vi "LV String to Str64.vi"(11 "string":string) -> (3 "str64":T1)   [LabVIEW 2026, in "MrcLib.lvlib"]
uses:
  MrcLib.lvlib
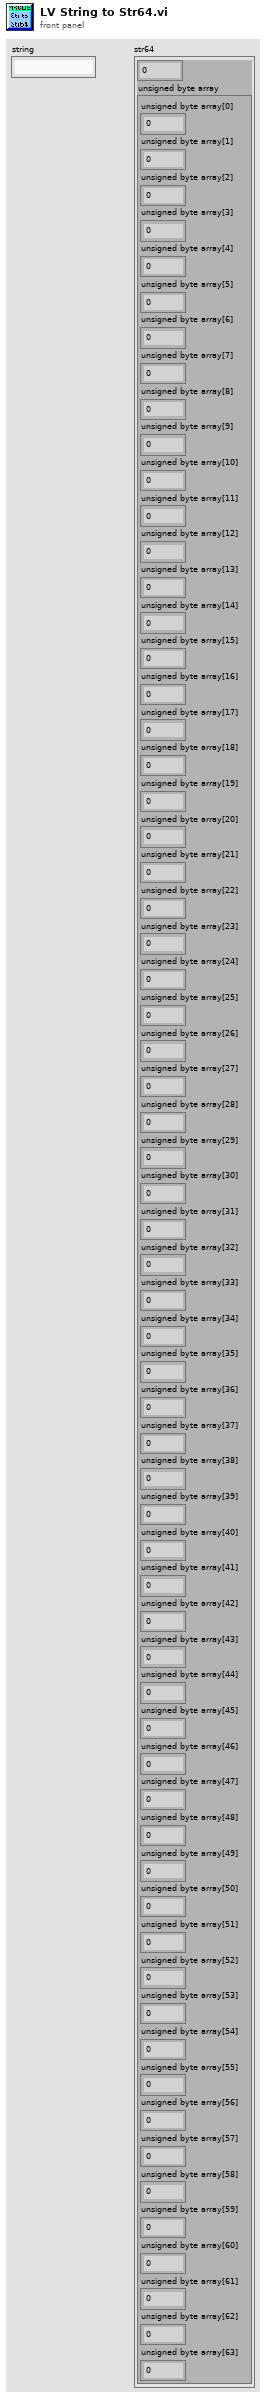
[diagram p1: front panel]
types:
  T1 = cluster{u8, "unsigned byte array":cluster{"unsigned byte array[0]":u8, "unsigned byte array[1]":u8, "unsigned byte array[2]":u8, "unsigned byte array[3]":u8, "unsigned byte array[4]":u8, "unsigned byte array[5]":u8, "unsigned byte array[6]":u8, "unsigned byte array[7]":u8, "unsigned byte array[8]":u8, "unsigned byte array[9]":u8, "unsigned byte array[10]":u8, "unsigned byte array[11]":u8, "unsigned byte array[12]":u8, "unsigned byte array[13]":u8, "unsigned byte array[14]":u8, "unsigned byte array[15]":u8, "unsigned byte array[16]":u8, "unsigned byte array[17]":u8, "unsigned byte array[18]":u8, "unsigned byte array[19]":u8, "unsigned byte array[20]":u8, "unsigned byte array[21]":u8, "unsigned byte array[22]":u8, "unsigned byte array[23]":u8, "unsigned byte array[24]":u8, "unsigned byte array[25]":u8, "unsigned byte array[26]":u8, "unsigned byte array[27]":u8, "unsigned byte array[28]":u8, "unsigned byte array[29]":u8, "unsigned byte array[30]":u8, "unsigned byte array[31]":u8, "unsigned byte array[32]":u8, "unsigned byte array[33]":u8, "unsigned byte array[34]":u8, "unsigned byte array[35]":u8, "unsigned byte array[36]":u8, "unsigned byte array[37]":u8, "unsigned byte array[38]":u8, "unsigned byte array[39]":u8, "unsigned byte array[40]":u8, "unsigned byte array[41]":u8, "unsigned byte array[42]":u8, "unsigned byte array[43]":u8, "unsigned byte array[44]":u8, "unsigned byte array[45]":u8, "unsigned byte array[46]":u8, "unsigned byte array[47]":u8, "unsigned byte array[48]":u8, "unsigned byte array[49]":u8, "unsigned byte array[50]":u8, "unsigned byte array[51]":u8, "unsigned byte array[52]":u8, "unsigned byte array[53]":u8, "unsigned byte array[54]":u8, "unsigned byte array[55]":u8, "unsigned byte array[56]":u8, "unsigned byte array[57]":u8, "unsigned byte array[58]":u8, "unsigned byte array[59]":u8, "unsigned byte array[60]":u8, "unsigned byte array[61]":u8, "unsigned byte array[62]":u8, "unsigned byte array[63]":u8}}
  T2 = cluster{"unsigned byte array[0]":u8, "unsigned byte array[1]":u8, "unsigned byte array[2]":u8, "unsigned byte array[3]":u8, "unsigned byte array[4]":u8, "unsigned byte array[5]":u8, "unsigned byte array[6]":u8, "unsigned byte array[7]":u8, "unsigned byte array[8]":u8, "unsigned byte array[9]":u8, "unsigned byte array[10]":u8, "unsigned byte array[11]":u8, "unsigned byte array[12]":u8, "unsigned byte array[13]":u8, "unsigned byte array[14]":u8, "unsigned byte array[15]":u8, "unsigned byte array[16]":u8, "unsigned byte array[17]":u8, "unsigned byte array[18]":u8, "unsigned byte array[19]":u8, "unsigned byte array[20]":u8, "unsigned byte array[21]":u8, "unsigned byte array[22]":u8, "unsigned byte array[23]":u8, "unsigned byte array[24]":u8, "unsigned byte array[25]":u8, "unsigned byte array[26]":u8, "unsigned byte array[27]":u8, "unsigned byte array[28]":u8, "unsigned byte array[29]":u8, "unsigned byte array[30]":u8, "unsigned byte array[31]":u8, "unsigned byte array[32]":u8, "unsigned byte array[33]":u8, "unsigned byte array[34]":u8, "unsigned byte array[35]":u8, "unsigned byte array[36]":u8, "unsigned byte array[37]":u8, "unsigned byte array[38]":u8, "unsigned byte array[39]":u8, "unsigned byte array[40]":u8, "unsigned byte array[41]":u8, "unsigned byte array[42]":u8, "unsigned byte array[43]":u8, "unsigned byte array[44]":u8, "unsigned byte array[45]":u8, "unsigned byte array[46]":u8, "unsigned byte array[47]":u8, "unsigned byte array[48]":u8, "unsigned byte array[49]":u8, "unsigned byte array[50]":u8, "unsigned byte array[51]":u8, "unsigned byte array[52]":u8, "unsigned byte array[53]":u8, "unsigned byte array[54]":u8, "unsigned byte array[55]":u8, "unsigned byte array[56]":u8, "unsigned byte array[57]":u8, "unsigned byte array[58]":u8, "unsigned byte array[59]":u8, "unsigned byte array[60]":u8, "unsigned byte array[61]":u8, "unsigned byte array[62]":u8, "unsigned byte array[63]":u8}
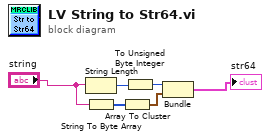
[diagram p0: block diagram]
diagram:
  n1 = String Length(string="string") -> (length=w1:i32)
  n2 = String To Byte Array(string="string") -> (unsigned byte array=w4:u8[])
  n3 = Array To Cluster(array=w4) -> (cluster=w5:T2)
  n4 = To Unsigned Byte Integer(number=w1) -> (unsigned 8bit integer=w6:u8)
  n5 = Bundle(w6, "unsigned byte array"=w5) -> (→"str64":T1)  [unwired: 1 in]
